vi "Hexapod_GUI.vi"(10 "stop 2":refnum<vi>, 11 "GUI_cluster":T1={"Sub Panel"=refnum, "GUIdevice"="Bella_LP_Mode", "CtlRef"=refnum, "User Event in"=refnum}) -> ()   [LabVIEW 2013]
uses:
  Shared/GUI_Template/GUI_master/tcp_new_data_event.ctl
  Shared/GUI_Template/GUI_master/tcp new data cluster.ctl
  Controls/GUI_cluster.ctl
  Controls/eventtypdef1.ctl
panel:
  in  "stepsize::1":dbl=0.02 caption="stepsize" min=0.0 max=10.0
  in  "<command>::1":bool=TRUE
  in  "stop":bool
  in  "wangle::1":dbl=0.19 caption="w" min=-5.0 max=5.0
  in  "vangle::1":dbl=0.0005 caption="v" min=-5.0 max=5.0
  in  "uangle::1":dbl=0.04 caption="u" min=-5.0 max=5.0
  in  "zpos::1":dbl=1.013 caption="z" min=-12.0 max=12.0
  in  "ypos::1":dbl=0.45 caption="y" min=-20.0 max=20.0
  in  "xpos::1":dbl=-1.0 caption="x" min=-20.0 max=20.0
  out "tcp data event":T2
  out "GUIdevice 1":string="StagingHexapodPI"
  in  "relativemove.yneg::1":bool caption="relativemove.ypos::1"
  in  "relativemove.xneg::1":bool caption="relativemove.xpos::1"
  in  "relativemove.ypos::1":bool caption="relativemove.yneg::1"
  in  "relativemove.xpos::1":bool caption="relativemove.xneg::1"
  in  "relativemove.zpos::1":bool
  in  "relativemove.zneg::1":bool
  in  "relativemove.wpos::1":bool
  in  "relativemove.uneg::1":bool caption="relativemove.upos::1"
  in  "relativemove.upos::1":bool caption="relativemove.uneg::1"
  in  "relativemove.vpos::1":bool
  in  "relativemove.vneg::1":bool
  in  "relativemove.wneg::1":bool
  # "+Z"
  # "+Y"
  # "-X"
  # "-Y"
  # "+X"
  # "-Z"
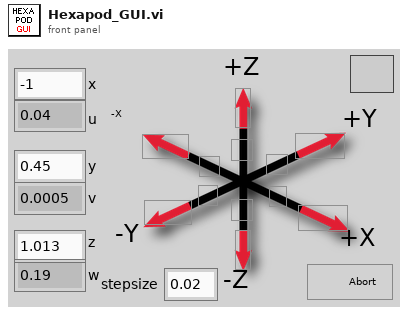
[diagram p1: front panel]
types:
  T1 = typedef "GUI_cluster.ctl" = cluster{"Sub Panel":refnum<vi>, "GUIdevice":string, "CtlRef":refnum<vi>, "User Event in":refnum<user-event>}
  T2 = typedef "tcp_new_data_event.ctl" = refnum<user-event>
  T3 = typedef "eventtypdef1.ctl" = cluster{"label":string, "Sub Panel":refnum<vi>, "CtlRef":refnum<vi>, "This VI":refnum<vi>}
  T4 = typedef "tcp new data cluster.ctl" = cluster{"EventEnum":enum16{"new data", "connection status update"}, "Device name":string}
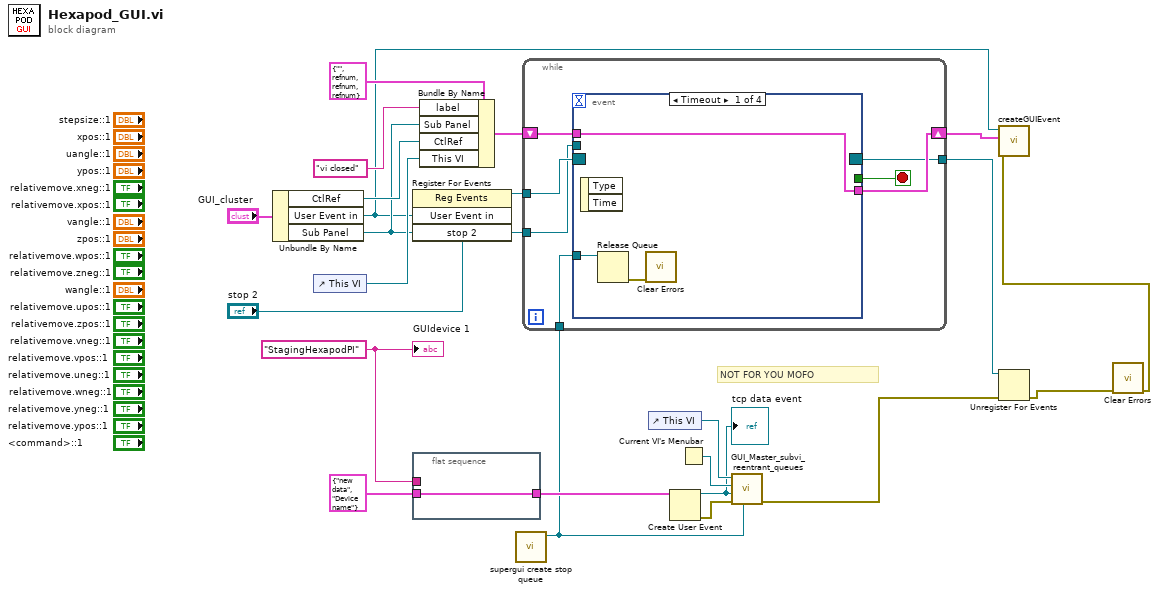
[diagram p0: block diagram]
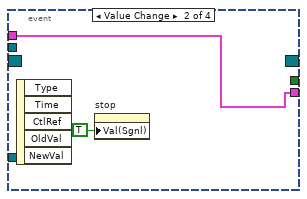
[diagram p2: hidden frame]
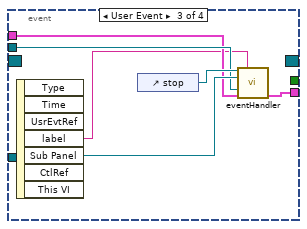
[diagram p3: hidden frame]
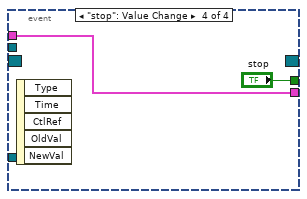
[diagram p4: hidden frame]
diagram:
  w13 = "StagingHexapodPI" ("GUIdevice")
  # "NOT FOR YOU MOFO"
  n1 = Unbundle By Name("GUI_cluster") -> ("CtlRef"=w15:refnum<vi>, "User Event in"=w8:refnum<user-event>, "Sub Panel"=w10:refnum<vi>)
  n2 = control-ref of="This VI"() -> (w14:refnum<vi>)
  n3 = register-events(w8, "stop 2") -> (reference out=w12:refnum<event-registration>)  [unwired: 2 in, 1 out]
  n4 = flat-sequence {
    tunnel: T4 {"EventEnum"=enum."new data", "Device name"="Device name"} ("New Event") -> [w24]
    tunnel: [w24] -> w16
    tunnel: w13 -> [_]
    frame #0 {
    }
  }
  n5 = Bundle By Name(cluster=T3 {"label"="", "Sub Panel"=refnum, "CtlRef"=refnum, "This VI"=refnum} ("event data"), "label"="vi closed", "Sub Panel"=w10, "CtlRef"=w15, "This VI"=w14) -> (w9:T3)
  n6 = call "supergui create stop queue.vi"() -> ("STOP Queue out"=w1:refnum<queue>)  [unwired: 11 in]
  n7 = while {
    tunnel: w12 -> [w31]
    tunnel: w10 -> [w29]
    shift-right: [w27] -> w7
    shift-left: w9 -> [w28]
    tunnel: [w26] -> w4
    tunnel: w1 -> [w25]
    stop <- w30 stop-if-true
    n8 = event shown="[0] Timeout" {
      selector: w31 -> [_ _ _ _]
      dyn-events: [_ _ _ _] -> w26
      timeout: _ -> [_ _ _ _]
      tunnel: [_ _ _ "stop"] -> w30
      tunnel: w29 -> [_ _ w40 _]
      tunnel: w28 -> [w34 w36 w39 w43]
      tunnel: [w34 w36 w38 w43] -> w27
      tunnel: w25 -> [w33 _ _ _]
      event Timeout {
        n9 = event-data() -> ()  [unwired: 1 in, 2 out]
        n10 = Release Queue(queue=w33) -> (error out=w32:errorcluster)  [unwired: 2 in, 2 out]
        n11 = call <vilib>:"Clear Errors.vi"("error in (no error)"=w32) -> ()  [unwired: 6 in, 1 out]
      }
      event Value Change {
        n12 = event-data() -> ()  [unwired: 1 in, 5 out]
        n13 = property on="stop" class="Bool (strict)"("Val(Sgnl)"=TRUE ("Value (Signaling)")) -> ()  [unwired: 2 in, 2 out]
      }
      event User Event {
        n14 = event-data() -> ("label"=w37:string, "Sub Panel"=w41:refnum<vi>)  [unwired: 1 in, 5 out]
        n15 = control-ref of="stop"() -> (w42:refnum<vi>)
        n16 = call "eventHandler.vi"("Boolean in"=w42, "label"=w37, "Sub Panel 2"=w41, "Sub Panel"=w40, "event data in"=w39) -> ("event data out"=w38:T3)  [unwired: 10 in]
      }
      event "stop": Value Change {
        n17 = event-data() -> ()  [unwired: 1 in, 5 out]
      }
    }
  }
  n18 = control-ref of="This VI"() -> (w23:refnum<vi>)
  n19 = Create User Event(user event datatype=w16) -> (user event=w20:refnum<user-event>, error out=w21:errorcluster)  [unwired: 1 in]
  "tcp data event" <- w20
  n20 = Current VI's Menubar() -> (w22:refnum<k9>)
  n21 = call "GUI_Master_subvi_reentrant_queues.vi"("STOP Queue in"=w1, "error in (no error)"=w21, "tcp data event"=w20, "Caller menu reference"=w22, "Caller VI ref"=w23) -> ("error out"=w3:errorcluster)  [unwired: 6 in]
  n22 = Unregister For Events(event registration refnum=w4, error in=w3) -> (error out=w5:errorcluster)
  n23 = call <vilib>:"Clear Errors.vi"("error in (no error)"=w5) -> ("error out"=w2:errorcluster)  [unwired: 6 in]
  n24 = call "createGUIEvent.vi"("error in (no error)"=w2, "event data"=w7, "User Event in"=w8) -> ()  [unwired: 8 in, 1 out]
  "GUIdevice 1" <- w13
